vi "JoystickToPoint.vi"(8 "Yw":dbl, 9 "Xw":dbl, 11 "JoystickIn":i32[](array[numeric])) -> (2 "y":dbl, 3 "x":dbl)   [LabVIEW 2013, in "ProcessorHelperFunctions.lvlib"]
uses:
  ProcessorHelperFunctions.lvlib
  <vilib>/Analysis/coordinate.llb/Angle Range (Degree).ctl
  <vilib>/Analysis/coordinate.llb/Angle Rotation (scalar).vi
  <vilib>/Analysis/coordinate.llb/Wrap Angle (scalar).vi
  <vilib>/Analysis/NI_AAL_Angle.lvlib
panel:
  in  "Mag Scaler":dbl=1.5
  # "Xw is x distance between the\nwheels on the robot"
  # "Yw is y distance between the\nwheels on the robot"
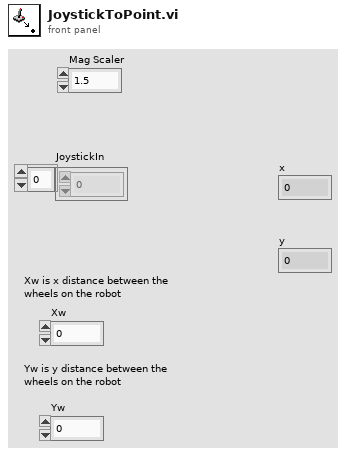
[diagram p1: front panel]
types:
  T1 = typedef "NI_AAL_Angle.lvlib/Angle Range (Degree).ctl" = u16
  T2 = cluster{"JoystickIn[0]":i32, "JoystickIn[1]":i32, "JoystickIn[2]":i32, "JoystickIn[3]":i32, "JoystickIn[4]":i32, "JoystickIn[5]":i32, "JoystickIn[6]":i32, "JoystickIn[7]":i32, "JoystickIn[8]":i32, "JoystickIn[9]":i32}
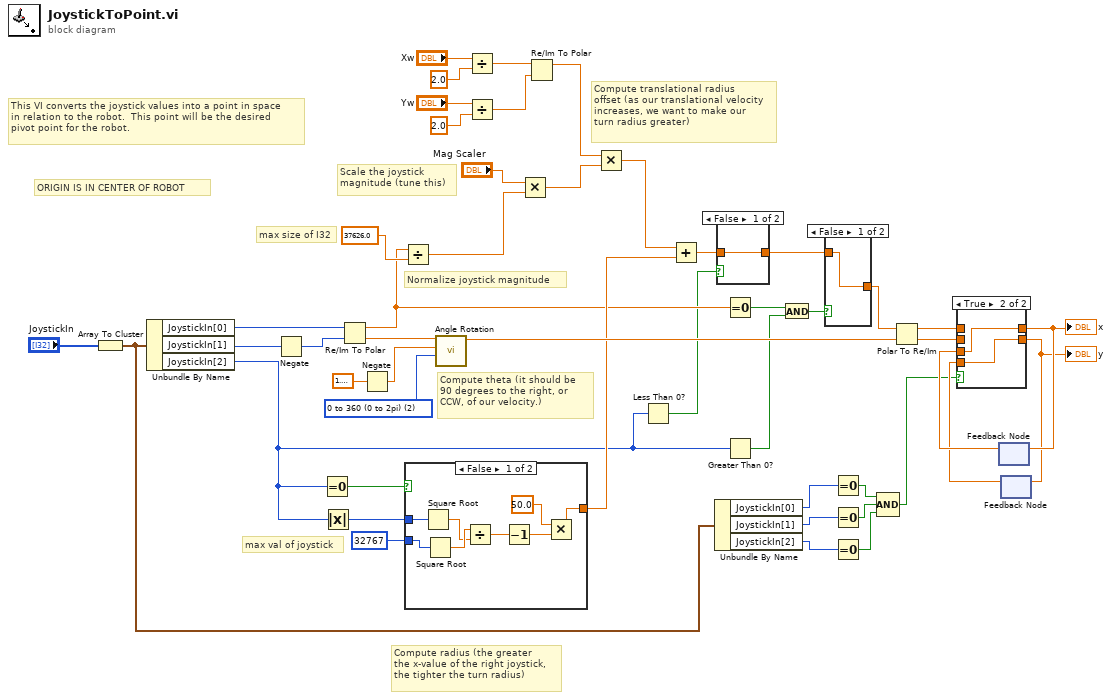
[diagram p0: block diagram]
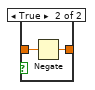
[diagram p3: hidden frame]
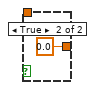
[diagram p4: hidden frame]
diagram:
  w44 = T1 2 items=["none", "-180 to 180 (-pi to pi)", "0 to 360 (0 to 2pi)"] ("rotated angle range")
  # "ORIGIN IS IN CENTER OF ROBOT"
  # "Scale the joystick\nmagnitude (tune this)"
  # "Compute theta (it should be \n90 degrees to the right, or \nCCW, of our velocity.)"
  # "Compute radius (the greater\nthe x-value of the right joystick,\nthe tighter the turn radius)"
  # "Compute translational radius \noffset (as our translational velocity\nincreases, we want to make our\nturn radius greater)"
  # "Normalize joystick magnitude"
  # "max size of I32"
  # "max val of joystick"
  # "This VI converts the joystick values into a point in space\nin relation to the robot.  This point will be the desired\npivot point for the robot."
  n1 = Array To Cluster(array="JoystickIn") -> (cluster=w14:T2)
  n2 = Unbundle By Name(w14) -> ("JoystickIn[0]"=w47:i32, "JoystickIn[1]"=w46:i32, "JoystickIn[2]"=w17:i32)
  n3 = Negate(x=w46) -> (-x=w15:i32)
  n4 = Equal To 0?(x=w17) -> (x = 0?=w42:bool)
  n5 = Absolute Value(x=w17) -> (abs(x)=w20:i32)
  n6 = Re/Im To Polar(2:w15, 3:w47) -> (0:w45:dbl, 1:w23:dbl)
  n7 = Negate(x=1.5707963267948966) -> (-x=w21:dbl)
  n8 = Divide(x=w23, y=37626.0) -> (x/y=w37:dbl)
  n9 = case shown="False" w42 {
    tunnel: 32767 -> [w55 w57]
    tunnel: w20 -> [w56 _]
    tunnel: [w51 w57] -> w33
    frame False {
      n10 = Square Root(x=w56) -> (sqrt(x)=w53:dbl)
      n11 = Square Root(x=w55) -> (sqrt(x)=w54:dbl)
      n12 = Divide(x=w54, y=w53) -> (x/y=w50:dbl)
      n13 = Decrement(x=w50) -> (x-1=w49:dbl)
      n14 = Multiply(x=50.0, y=w49) -> (x*y=w51:dbl)
    }
    frame True {
    }
  }
  n15 = call-poly <vilib>:"Angle Rotation.vi"("rotated angle range"=w44, "counterclockwise rotation"=w21, "angle"=w45) -> ("rotated angle"=w40:dbl)  [unwired: 7 in, 1 out]
  n16 = Divide(x="Xw", y=2.0) -> (x/y=w28:dbl)
  n17 = Divide(x="Yw", y=2.0) -> (x/y=w27:dbl)
  n18 = Multiply(x="Mag Scaler", y=w37) -> (x*y=w36:dbl)
  n19 = Re/Im To Polar(2:w27, 3:w28) -> (1:w35:dbl)  [unwired: 1 out]
  n20 = Multiply(x=w35, y=w36) -> (x*y=w34:dbl)
  n21 = Less Than 0?(x=w17) -> (x < 0?=w16:bool)
  n22 = Add(x=w34, y=w33) -> (x+y=w19:dbl)
  n23 = Unbundle By Name(w14) -> ("JoystickIn[0]"=w13:i32, "JoystickIn[1]"=w12:i32, "JoystickIn[2]"=w11:i32)
  n24 = case shown="False" w16 {
    tunnel: w19 -> [w58 w60]
    tunnel: [w58 w59] -> w18
    frame False {
    }
    frame True {
      n25 = Negate(x=w60) -> (-x=w59:dbl)
    }
  }
  n26 = Equal To 0?(x=w23) -> (x = 0?=w24:bool)
  n27 = Greater Than 0?(x=w17) -> (x > 0?=w25:bool)
  n28 = And(x=w24, y=w25) -> (x .and. y?=w26:bool)
  n29 = case shown="False" w26 {
    tunnel: w18 -> [w61 _]
    tunnel: [w61 0.0] -> w22
    frame False {
    }
    frame True {
    }
  }
  n30 = Equal To 0?(x=w13) -> (x = 0?=w10:bool)
  n31 = Equal To 0?(x=w12) -> (x = 0?=w9:bool)
  n32 = Equal To 0?(x=w11) -> (x = 0?=w8:bool)
  n33 = Compound Arithmetic op=AND(w10, w9, w8) -> (w1:bool)
  n34 = Polar To Re/Im(2:w40, 3:w22) -> (0:w5:dbl, 1:w7:dbl)
  n35 = feedback #1() -> (w3:dbl)  [unwired: 1 in]
  n36 = feedback #2() -> (w2:dbl)  [unwired: 1 in]
  n37 = case shown="True" w1 {
    tunnel: w7 -> [w64 _]
    tunnel: [w64 w66] -> w6
    tunnel: w5 -> [w63 _]
    tunnel: [w63 w65] -> w4
    tunnel: w3 -> [_ w66]
    tunnel: w2 -> [_ w65]
    frame False {
    }
    frame True {
    }
  }
  "x" <- w6
  "y" <- w4
  n38 = feedback-in #1(w6) -> ()
  n39 = feedback-in #2(w4) -> ()
